vi "Init.vi"(8 "error in (no error)":errorcluster, 11 "TileTimer in":refnum<class "TileTimer.lvclass">) -> (0 "error out":errorcluster, 3 "TileTimer out":refnum<class "TileTimer.lvclass">)   [LabVIEW 2019, in "RT_Game.lvlib" / "TileTimer.lvclass"]
uses:
  TileTimer.lvclass
  GameObject/GameObject.lvclass
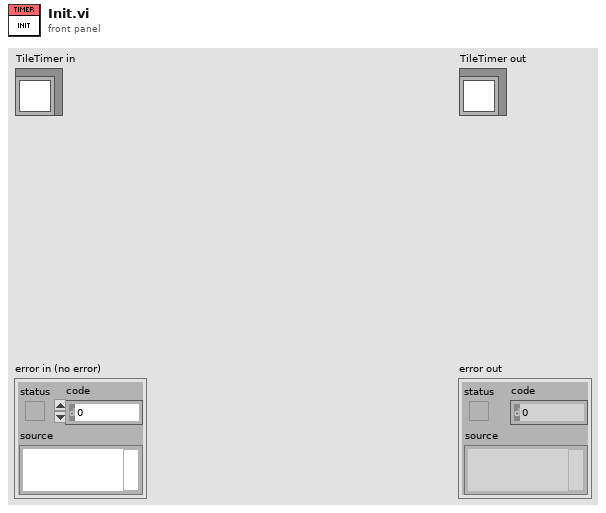
[diagram p1: front panel]
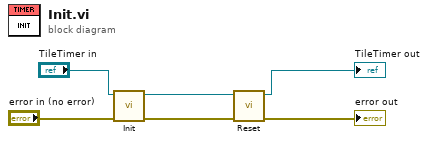
[diagram p0: block diagram]
diagram:
  n1 = call-parent "Init.vi"("error in (no error)"="error in (no error)", "GameObject in"="TileTimer in") -> ("error out"=w6:errorcluster, "GameObject out"=w2:refnum<class "TileTimer.lvclass">)  [unwired: 8 in]
  n2 = call "Reset.vi"("error in (no error)"=w6, "TileTimer in"=w2) -> ("error out"=→"error out":errorcluster, "TileTimer out"=→"TileTimer out":refnum<class "TileTimer.lvclass">)  [unwired: 8 in]
